vi "Fit Peaks.vi"(8 "error in (no error)":errorcluster, 10 "Y":dbl[](array[numeric]), 11 "Ocean Optics Driver in":refnum<class "Ocean Optics Driver.lvclass">) -> (0 "error out":errorcluster, 3 "Ocean Optics Driver out":refnum<class "Ocean Optics Driver.lvclass">)   [LabVIEW 2016, in "Ocean Optics Driver.lvclass"]
uses:
  Ocean Optics Driver.lvclass
  C:/github/NHMFL_Core/Libraries/Instruments/Spectrometer Driver/Spectrometer Driver.lvclass
  Spectrometer Driver/Spectrometer Driver.lvclass/Spectrometer Driver.ctl
  Ocean Optics Driver.lvclass/Ocean Optics Driver.ctl
  Spectrometer Driver/Read Wavelengths.vi
  Spectrometer Driver/Write Peaks.vi
  Read Ocean optics configuration.vi
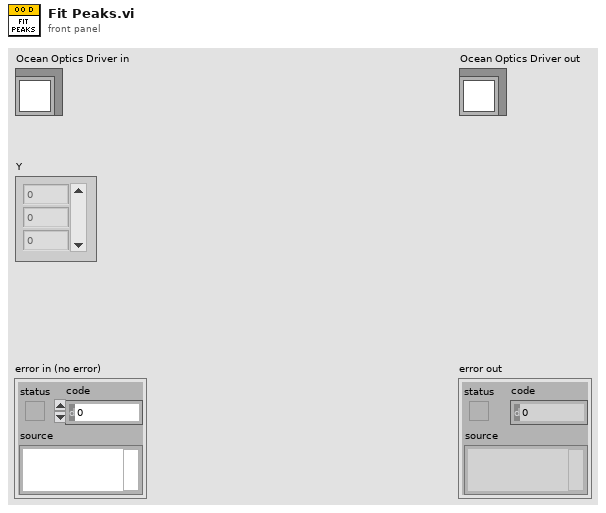
[diagram p1: front panel]
types:
  T1 = typedef "Ruby Spectra.lvclass/Ocean optics configuration.ctl" = cluster{"Integration time":dbl, "Fit parameters":T2, "Fit":bool, "Auto-update params":bool, "Save spectra":bool, "Reference wavelengh":dbl, "Background":path}
  T2 = typedef "Multi-peak Parameters.ctl" = cluster{"Function":enum16{"Gauss", "Lorentz"}, "Window width":dbl, "Initial guess":T3}
  T3 = typedef "Peak Parameters.ctl" = cluster{"Amplitude":dbl, "Center":dbl, "Width":dbl}
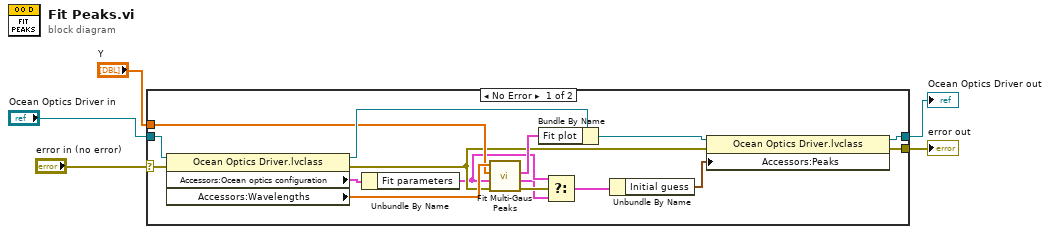
[diagram p0: block diagram]
diagram:
  n1 = case shown="No Error" "error in (no error)" {
    selector: "error in (no error)" -> [w21 w23]
    tunnel: [w14 w23] -> w4
    tunnel: [w12 w22] -> w2
    tunnel: "Ocean Optics Driver in" -> [w20 w22]
    tunnel: "Y" -> [w16 _]
    frame No Error {
      n2 = property class="Ocean Optics Driver.lvclass"(reference=w20, error in=w21) -> (reference out=w19:refnum<class "Ocean Optics Driver.lvclass">, error out=w9:errorcluster, "Accessors:Ocean optics configuration"=w18:T1, "Accessors:Wavelengths"=w17:dbl[])
      n3 = Unbundle By Name(w18) -> ("Fit parameters"=w8:T2)
      n4 = call "Fit Multi-Gaus Peaks.vi"("Error In"=w9, "Fit parameters"=w8, "Y"=w16, "X"=w17) -> ("Error Out"=w10:errorcluster, "Fit parameters out"=w7:T2, "Fit plot"=w15:cluster{"Array":dbl[], "Array":dbl[]})  [unwired: 5 in]
      n5 = Bundle By Name(cluster=w19, "Fit plot"=w15) -> (w13:refnum<class "Ocean Optics Driver.lvclass">)
      n6 = Select(t=w8, s=w10, f=w7) -> (s? t:f=w6:T2)
      n7 = Unbundle By Name(w6) -> ("Initial guess"=w11:T3)
      n8 = property class="Ocean Optics Driver.lvclass"(reference=w13, error in=w9, "Accessors:Peaks"=w11) -> (reference out=w12:refnum<class "Ocean Optics Driver.lvclass">, error out=w14:errorcluster)
    }
    frame Error {
    }
  }
  "error out" <- w4
  "Ocean Optics Driver out" <- w2
